vi "updateInicatorsMainVi.vi"(6 "Data String out":string, 7 "Boolean":bool, 9 "Array":refnum<vi>[](array[refnum]), 10 "Channel Selector":string, 11 "error in":errorcluster) -> (0 "Data String out 2":string, 3 "error out":errorcluster)   [LabVIEW 2013]
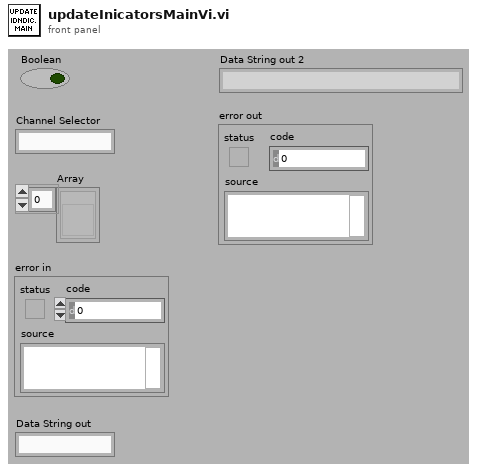
[diagram p1: front panel]
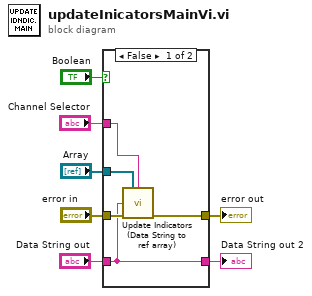
[diagram p0: block diagram]
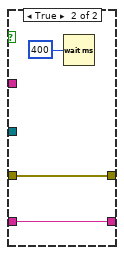
[diagram p2: hidden frame]
diagram:
  n1 = case shown="False" "Boolean" {
    tunnel: "Array" -> [w11 _]
    tunnel: "error in" -> [w10 w15]
    tunnel: [w12 w15] -> w2
    tunnel: "Channel Selector" -> [w8 _]
    tunnel: [w9 w13] -> w5
    tunnel: "Data String out" -> [w9 w13]
    frame False {
      n2 = call "Update Indicators (Data String to ref array).vi"("Array"=w11, "Active Channel"=w8, "Data String"=w9, "error in (no error)"=w10) -> ("error out"=w12:errorcluster)  [unwired: 10 in, 1 out]
    }
    frame True {
      n3 = Wait (ms)(milliseconds to wait=u32 400) -> ()  [unwired: 1 out]
    }
  }
  "Data String out 2" <- w5
  "error out" <- w2
